vi "SaveReadImage.vi"() -> ()   [LabVIEW 2014]
uses:
  <vilib>/picture/picture.llb/imagedata.ctl
  <vilib>/picture/picture.llb/Draw True-Color Pixmap.vi
panel:
  out "Color 256":T1
  out "new picture":picture
  out "new picture 2":picture
  out "error out":errorcluster
  in  "file path":path
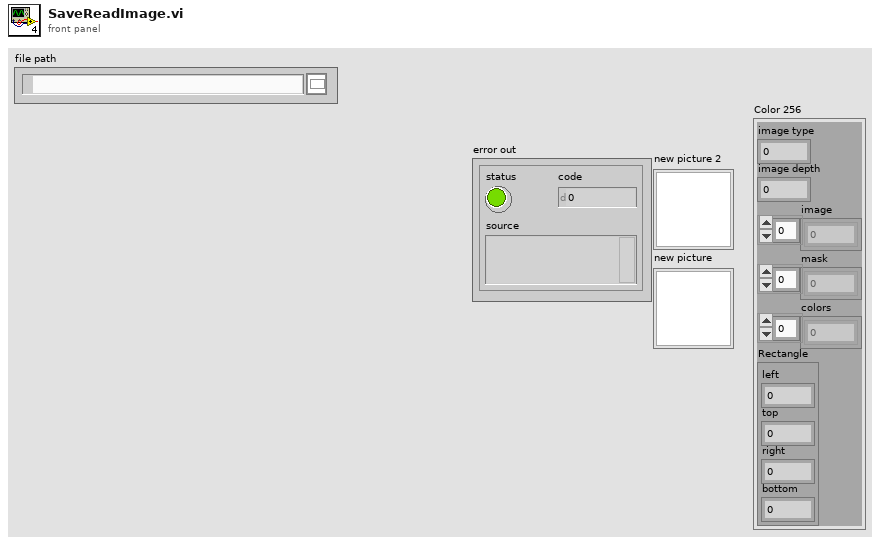
[diagram p1: front panel]
types:
  T1 = typedef "imagedata.ctl" = cluster{"image type":i32, "image depth":i32, "image":u8[], "mask":u8[], "colors":u32[], "Rectangle":cluster{"left":i16, "top":i16, "right":i16, "bottom":i16}}
  T2 = enum16{"open", "open or create", "create or replace", "create", "open (read-only)"}
  T3 = cluster{"left":i16, "top":i16, "right":i16, "bottom":i16}
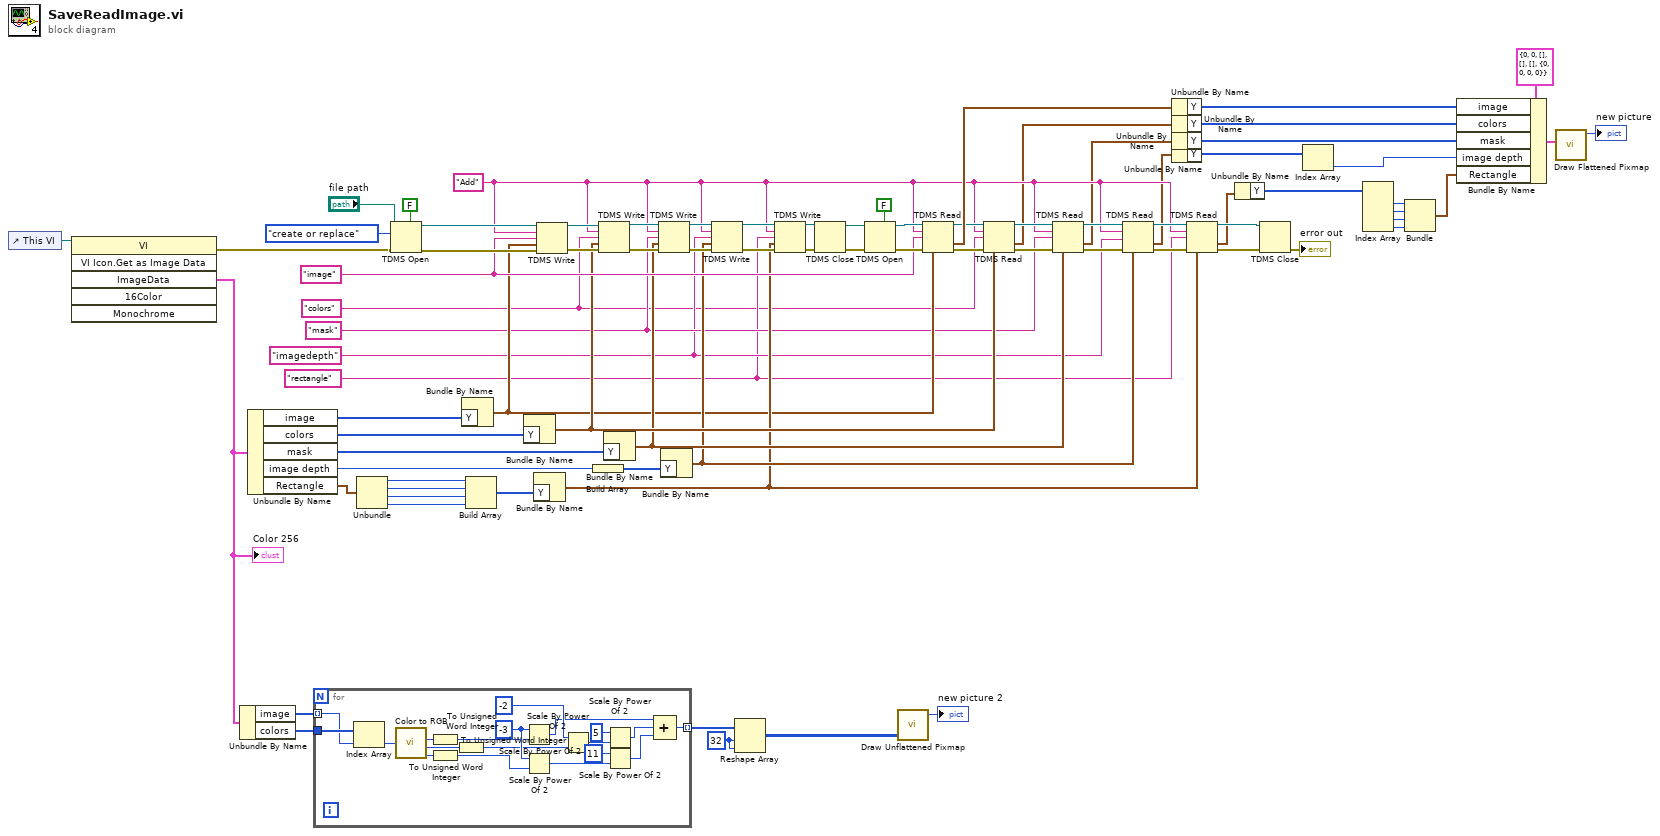
[diagram p0: block diagram]
diagram:
  w5 = "rectangle" ("group name in (Untitled)")
  w6 = "imagedepth" ("group name in (Untitled)")
  w7 = "mask" ("group name in (Untitled)")
  w4 = "colors" ("group name in (Untitled)")
  w63 = 32 ("dimension size")
  w71 = "image" ("group name in (Untitled)")
  w31 = "Add" ("group name in (Untitled)")
  n1 = control-ref of="This VI"() -> (w2:refnum<vi>)
  n2 = invoke class="VI" method="VI Icon.Get as Image Data"(reference=w2) -> (error out=w3:errorcluster, "ImageData"=w62:T1)  [unwired: 5 in, 4 out]
  "Color 256" <- w62
  n3 = Unbundle By Name(w62) -> ("image"=w66:u8[], "colors"=w65:u32[])
  n4 = Unbundle By Name(w62) -> ("image"=w68:u8[], "colors"=w58:u32[], "mask"=w57:u8[], "image depth"=w56:i32, "Rectangle"=w1:T3)
  n5 = for {
    tunnel: w66 -> [w99] mode=indexing
    tunnel: w65 -> [w100]
    tunnel: [w84] -> w64 mode=indexing
    w97 = i16 -3 ("n")
    n6 = Index Array(array=w100, index=w99) -> (element=w98:u32)
    n7 = call <vilib>:"Color to RGB.vi"("Color"=w98) -> ("R"=w93:u8, "G"=w92:u8, "B"=w90:u8)  [unwired: 1 out]
    n8 = To Unsigned Word Integer(number=w93) -> (unsigned 16bit integer=w82:u16)
    n9 = To Unsigned Word Integer(number=w90) -> (unsigned 16bit integer=w83:u16)
    n10 = To Unsigned Word Integer(number=w92) -> (unsigned 16bit integer=w91:u16)
    n11 = Scale By Power Of 2(n=w97, x=w82) -> (x*2^n=w87:u16)
    n12 = Scale By Power Of 2(n=w97, x=w83) -> (x*2^n=w89:u16)
    n13 = Scale By Power Of 2(n=i16 -2, x=w91) -> (x*2^n=w95:u16)
    n14 = Scale By Power Of 2(n=i16 5, x=w95) -> (x*2^n=w86:u16)
    n15 = Scale By Power Of 2(n=i16 11, x=w89) -> (x*2^n=w85:u16)
    n16 = Compound Arithmetic op=ADD(w87, w86, w85) -> (w84:u16)
  }
  n17 = Unbundle(w1) -> ("left"=w54:i16, "top"=w53:i16, "right"=w52:i16, "bottom"=w51:i16)
  n18 = TDMS Open(5:FALSE ("create index file? (T)"), 8:w3, 10:T2."create or replace" ("operation (0:open)"), 11:"file path") -> (0:w75:errorcluster, 3:w76:refnum<k34>)  [unwired: 3 in]
  n19 = Bundle By Name("Y"=w68) -> (w12:waveform(u8))  [unwired: 1 in]
  n20 = Build Array(w54, w53, w52, w51) -> (w50:i16[])
  n21 = Bundle By Name("Y"=w58) -> (w23:waveform(u32))  [unwired: 1 in]
  n22 = Bundle By Name("Y"=w50) -> (w20:waveform(i16))  [unwired: 1 in]
  n23 = TDMS Write(0:w76, 5:w31, 7:w71, 9:w12, 11:w75) -> (4:w60:refnum<k34>, 15:w59:errorcluster)  [unwired: 1 in, 2 out]
  n24 = Build Array(w56) -> (w55:i32[])
  n25 = TDMS Write(0:w60, 5:w31, 7:w4, 9:w23, 11:w59) -> (4:w49:refnum<k34>, 15:w46:errorcluster)  [unwired: 1 in, 2 out]
  n26 = Bundle By Name("Y"=w57) -> (w22:waveform(u8))  [unwired: 1 in]
  n27 = TDMS Write(0:w49, 5:w31, 7:w7, 9:w22, 11:w46) -> (4:w48:refnum<k34>, 15:w47:errorcluster)  [unwired: 1 in, 2 out]
  n28 = Bundle By Name("Y"=w55) -> (w21:waveform(i32))  [unwired: 1 in]
  n29 = TDMS Write(0:w48, 5:w31, 7:w6, 9:w21, 11:w47) -> (4:w45:refnum<k34>, 15:w42:errorcluster)  [unwired: 1 in, 2 out]
  n30 = Reshape Array(w64, w63, w63) -> (w61:u16[][])
  n31 = TDMS Write(0:w45, 5:w31, 7:w5, 9:w20, 11:w42) -> (4:w44:refnum<k34>, 15:w43:errorcluster)  [unwired: 1 in, 2 out]
  n32 = TDMS Close(8:w43, 11:w44) -> (0:w81:errorcluster, 3:w80:path)
  n33 = TDMS Open(5:FALSE ("create index file? (T)"), 8:w81, 11:w80) -> (0:w73:errorcluster, 3:w74:refnum<k34>)  [unwired: 4 in]
  n34 = call-poly <vilib>:"Draw Unflattened Pixmap.vi"("data (RGB format)"=w61) -> ("new picture"=→"new picture 2":picture)  [unwired: 8 in]
  n35 = TDMS Read(0:w74, 5:w31, 7:w71, 11:w73, 12:w12) -> (4:w41:refnum<k34>, 10:w72:waveform(u8), 15:w32:errorcluster)  [unwired: 3 in, 3 out]
  n36 = TDMS Read(0:w41, 5:w31, 7:w4, 11:w32, 12:w23) -> (4:w40:refnum<k34>, 10:w30:waveform(u32), 15:w33:errorcluster)  [unwired: 3 in, 3 out]
  n37 = TDMS Read(0:w40, 5:w31, 7:w7, 11:w33, 12:w22) -> (4:w39:refnum<k34>, 10:w29:waveform(u8), 15:w34:errorcluster)  [unwired: 3 in, 3 out]
  n38 = TDMS Read(0:w39, 5:w31, 7:w6, 11:w34, 12:w21) -> (4:w38:refnum<k34>, 10:w28:waveform(i32), 15:w35:errorcluster)  [unwired: 3 in, 3 out]
  n39 = Unbundle By Name(w72) -> ("Y"=w19:u8[])
  n40 = Unbundle By Name(w30) -> ("Y"=w25:u32[])
  n41 = Unbundle By Name(w29) -> ("Y"=w24:u8[])
  n42 = Unbundle By Name(w28) -> ("Y"=w11:i32[])
  n43 = TDMS Read(0:w38, 5:w31, 7:w5, 11:w35, 12:w20) -> (4:w37:refnum<k34>, 10:w27:waveform(i16), 15:w36:errorcluster)  [unwired: 3 in, 3 out]
  n44 = Unbundle By Name(w27) -> ("Y"=w18:i16[])
  n45 = TDMS Close(8:w36, 11:w37) -> (0:→"error out":errorcluster)  [unwired: 1 out]
  n46 = Index Array(array=w11) -> (element=w10:i32)  [unwired: 1 in]
  n47 = Index Array(array=w18) -> (element #1=w17:i16, element #2=w16:i16, element #3=w15:i16, element #4=w14:i16)  [unwired: 4 in]
  n48 = Bundle(w17, w16, w15, w14) -> (w13:cluster{i16, i16, i16, i16})  [unwired: 1 in]
  n49 = Bundle By Name(cluster=T1 {"image type"=0, "image depth"=0, "image"=[], "mask"=[], "colors"=[], "Rectangle"={"left"=0, "top"=0, "right"=0, "bottom"=0}} ("Color 256"), "image"=w19, "colors"=w25, "mask"=w24, "image depth"=w10, "Rectangle"=w13) -> (w9:T1)
  n50 = call <vilib>:"Draw Flattened Pixmap.vi"("image data"=w9) -> ("new picture"=→"new picture":picture)  [unwired: 8 in]
